vi "InitializeInstrument.vi"(8 "error in (no error)":errorcluster, 11 "reference in":refnum<class "niMmWave_Transceiver.lvclass">) -> (0 "error out":errorcluster, 3 "reference out":refnum<class "niMmWave_Transceiver.lvclass">)   [LabVIEW 2019, in "niMmWave_Transceiver.lvclass"]
doc: "Opens instrument session(s) and performs initial configuration for selected mode.\n\nInputs:\n<b>Initialization source</b> ini file and ini section to be read\n<b>Mode</b> specifies operation mode: BB/IF/RF"
uses:
  niMmWave_Transceiver.lvclass
  C:/Barkhausen mmWave radar/Development/modules/mmw_instrument/src_LabVIEW/Host/SubVIs/mmWave instrument_class/mmWave instrument.lvclass
  Low-level/TypeDefs/Resources.ctl
  <vilib>/userdefined/High Color/nirio_resource_hc.ctl
  mmWave instrument_class/Instrument state.ctl
  Low-level/TypeDefs/Hardware Configuration.ctl
  Low-level/TypeDefs/Direction.ctl
  mmWave HW Control/mmWave HW Control.lvlib
  mmWave instrument_class/mmWave instrument.lvclass
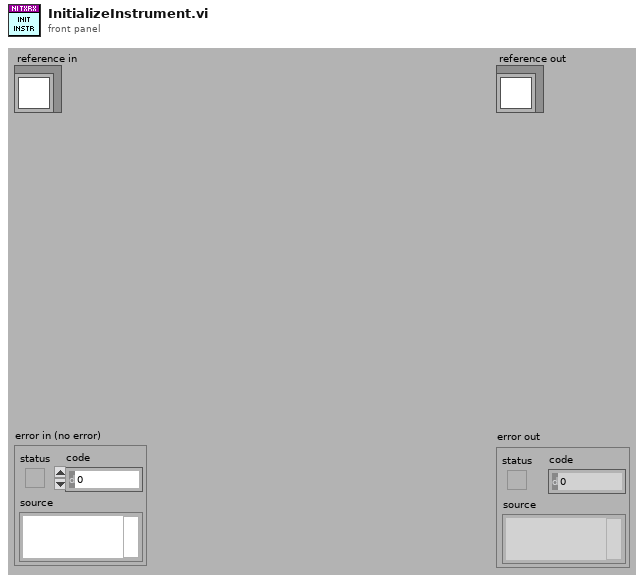
[diagram p1: front panel]
types:
  T1 = typedef "mmWave instrument.lvclass/Instrument state.ctl" = enum16{"Off", "Initialization", "Configuration", "Running", "Calibration"}
  T2 = typedef "Resources.ctl" = cluster{"7902R (Tx)":T3, "3610 (Tx)":refnum<visa-resource-name>, "3620 (IF)":T3, "3630 (RX)":refnum<visa-resource-name>, "7902R (Rx)":T3}
  T3 = typedef "nirio_resource_hc.ctl" = tag
  T4 = typedef "mmWave instrument.lvclass/ObjectAttributesRef.ctl" = refnum<data-value>
  T5 = typedef "niMmWave_Transceiver.lvclass/ObjectAttributesRef.ctl" = refnum<data-value>
  T6 = typedef "niMmWave_Transceiver.lvclass/ObjectAttributes.ctl" = cluster{"session":T7[], "HW.RX resources":T21, "RF config":T22, "RX trigger options":T23, "TX trigger options":T23, "RX samples":i32, "Downloaded Bursts":map{string, T26}, "TX Fs":dbl, "RX Fs":dbl, "burst sequence":string[]}
  T7 = typedef "Session.ctl" = cluster{"3620 session":refnum<queue>, "tx baseband session":T8, "rx baseband session":T16, "tx gain (dB)":dbl, "rx gain (dB)":dbl, "hardware configuration":T17, "gain ranging":T19[], "pxi trigger bus information":T20}
  T8 = typedef "Tx Baseband Session.ctl" = cluster{"3610 session":T9, "7902 reference":T15}
  T9 = typedef "ni3610_and_ni3630_Driver_Lib.lvlib/Main Settings.ctl" = cluster{"VISA resource name":refnum<visa-resource-name>, "Address Space":T10, "window_offset":u32, "register_addresses":T11, "required_MM_fpga_version":cluster{"signature":u32, "hardware":u32, "current revision":u32, "oldest revision":u32}, "CPLD Oldest Compat Version ":cluster{"hardware":u32, "CPLD firmware":u32}, "MM_FPGA_image_location":string, "is_init":bool, "card_type":T12, "DacLmkConfigFileName":string, "AdcLmkConfigFileName":string, "AdcConfigFileName":string, "DacConfigFileName_RevA":string, "DacConfigFileName_RevB":string, "Mulde hardware revision":u8, "bypass DAC PLL\n":bool, "IQ Card Revision":T13, "board capability":T14}
  T10 = typedef "VISA Register Access Address Space.ctl" = u16
  T11 = typedef "ni3610_and_ni3630_Driver_Lib.lvlib/Register Adresses.ctl" = cluster{"MM based Registers":cluster{"Revision":u32, "OldestCompatRev":u32, "signature":u32, "scratch":u32, "LedControl":u32, "BoardHwRev":u32, "BoardControl":u32, "ThermalStatus":u32, "BasebandStatus":u32, "BasebandControl":u32, "BasebandAuxSetup":u32, "BasebandAuxStatus":u32, "LmkSyncOutSetup":u32, " AdcSyncOutSetup":u32, " InjSyncOutSetup":u32, " PxiTrig0OutSetup":u32, " PxiTrig1OutSetup":u32, " PxiTrig2OutSetup":u32, " PxiTrig3OutSetup":u32, " PxiTrig4OutSetup":u32, " PxiTrig5OutSetup":u32, " PxiTrig6OutSetup":u32, " PxiTrig7OutSetup":u32}, "CPLD based Registers":cluster{"SlaveSignature":u32, "SlaveRevision":u32, "SlaveOldestCompatRev":u32, "SlaveScratch":u32, "SlaveSetup":u32, "SlaveStatus":u32, "IDacReg_offset":u32, "LMKRegGrp0_offset":u32, "QDacReg_offset":u32, "BrdTempSensorVal":u32, "TempSensorPowerDown":u32, "GPIOReg_offset":u32, "IAdcReg_offset":u32, "QAdcReg_offset":u32, "LMKRegGrp1_offset":u32, "QadcTempSensorVal":u32, "IadcTempSensorVal":u32, "RevisionReg":u32, "VcxoReg":u32, "CpldStatusReg":u32, "PowerReg":u32, "VBiasEnReg":u32, "ExtRefOeReg":u32, "QdacCtrlReg":u32, "QdacStatusReg":u32, "IdacCtrlReg":u32, "IdacStatusReg":u32, "QdacJtagIn":u32, "QdacJtagOut":u32, "IdacJtagIn":u32, "IdacJtagOut":u32, "IqDcSetupReg":u32, "QadcStatusReg":u32, "IadcStatusReg":u32, "BrdSetupReg":u32, "IqDcRevisionReg":u32, "PllStatusReg":u32, "EndpointScratchReg":u32, "AdcSyncCfgReg":u32, "IqCardOpampReg":u32}, "CPLD Register Offset":u32, "MM  Register Offset":u32, " PxiTrig0OutSetup":u32}
  T12 = typedef "ni3610_and_ni3630_Driver_Lib.lvlib/Base Card Type.ctl" = enum16{"unspecified", "ADC", "DAC"}
  T13 = typedef "ni3610_and_ni3630_Driver_Lib.lvlib/IQ Card Revision.ctl" = enum16{"RevA", "RevB", "RevC", "RevD"}
  T14 = typedef "ni3610_and_ni3630_Driver_Lib.lvlib/Board Capability.ctl" = cluster{"baseband sync":enum16{"no baseband sync", "baseband sync"}}
  T15 = typedef "Blank FPGA Reference.ctl" = refnum<k20>
  T16 = typedef "Rx Baseband Session.ctl" = cluster{"3630 session":T9, "7902 reference":T15}
  T17 = typedef "Hardware Configuration.ctl" = cluster{"direction":T18, "baseband only":bool}
  T18 = typedef "Direction.ctl" = enum16{"Transceiver", "Receiver", "Transmitter"}
  T19 = typedef "Gain Ranging.ctl" = cluster{"gain ranging active scope":string, "gain ranging stream session":refnum<k20>}
  T20 = typedef "PXI Trigger Bus Info.ctl" = cluster{"chassis resource name":refnum<visa-resource-name>, "7902R (TX)":i16, "3610 (TX)":i16, "3620 (IF)":i16, "3630 (RX)":i16, "7902R (RX)":i16}
  T21 = typedef "mmWave HW Control.lvlib/HW TXRX resources cluster.ctl" = cluster{"TX_DAC":refnum<visa-resource-name>, "TX_FPGA":tag, "IF":tag, "RX_ADC":refnum<visa-resource-name>, "RX_FPGA":tag}
  T22 = typedef "mmWave HW Control.lvlib/HW TXRX RF config cluster.ctl" = cluster{"TX.Frequency":dbl, "TX.Gain":dbl, "TX.mmWave adapter":string, "RX.Frequency":dbl, "RX.Gain":dbl, "RX.mmWave adapter":string}
  T23 = typedef "TX trigger config.ctl" = cluster{"delay":dbl, "trig source":T24, "PXI src":i32, "export":T25, "PXI dest":i32}
  T24 = typedef "FPGA Utility.lvlib/FPGA driver trigger source.ctl" = enum16{"Use Tclk", "PXI_Trig", "Aurora RX trig"}
  T25 = typedef "FPGA Utility.lvlib/FPGA driver trigger destination.ctl" = enum16{"None", "Source trig", "Synced trig", "Delayed sync"}
  T26 = typedef "niMmWave_Transceiver.lvclass/BurstInfo.ctl" = cluster{"starting addr":u32, "end addr":u32}
  T27 = typedef "mmWave instrument.lvclass/ObjectAttributes.ctl" = cluster{"mode":T28, "instr state":T1, "Max Fs":dbl, "Equalization coeff":cdb[], "LO sync en":bool, "Trig sync en":bool, "LO sources":T29, "LO Export":T30, "Fc.range":cluster{"min":dbl, "max":dbl}, "Sync mode":T31, "equalization en":bool, "sequence":string[]}
  T28 = typedef "mmWave instrument.lvclass/Instrument mode.ctl" = enum16{"RF", "IF", "BB"}
  T29 = typedef "mmWave HW Control.lvlib/LO sources.ctl" = cluster{"RX/LO1 src":string, "TX/LO1 src":string, "LO2 src":string}
  T30 = typedef "mmWave HW Control.lvlib/LO export.ctl" = cluster{"TX LO1 export":bool, "TX LO1 export level":dbl, "RX LO1 export":bool, "RX LO1 export level":dbl, "LO2 export":bool, "LO2 export level":dbl}
  T31 = typedef "mmWave instrument.lvclass/Sync mode.ctl" = enum16{"Slave", "Master"}
  T32 = typedef "Detected mmWave Adapters.ctl" = cluster{"3620 resource name":T3, "detected mmWave adapters":T33[]}
  T33 = typedef "mmWave Adapter Information.ctl" = cluster{"scope":string, "mmWave adapter type":string, "serial number":u64}
  T34 = typedef "Constants.ctl" = cluster{"data clock rate (Hz)":dbl, "sample rate (Hz)":dbl, "sample rate selector string":string, "default tx bitfile path":path, "default rx bitfile path":path, "default proc bitfile path":path}
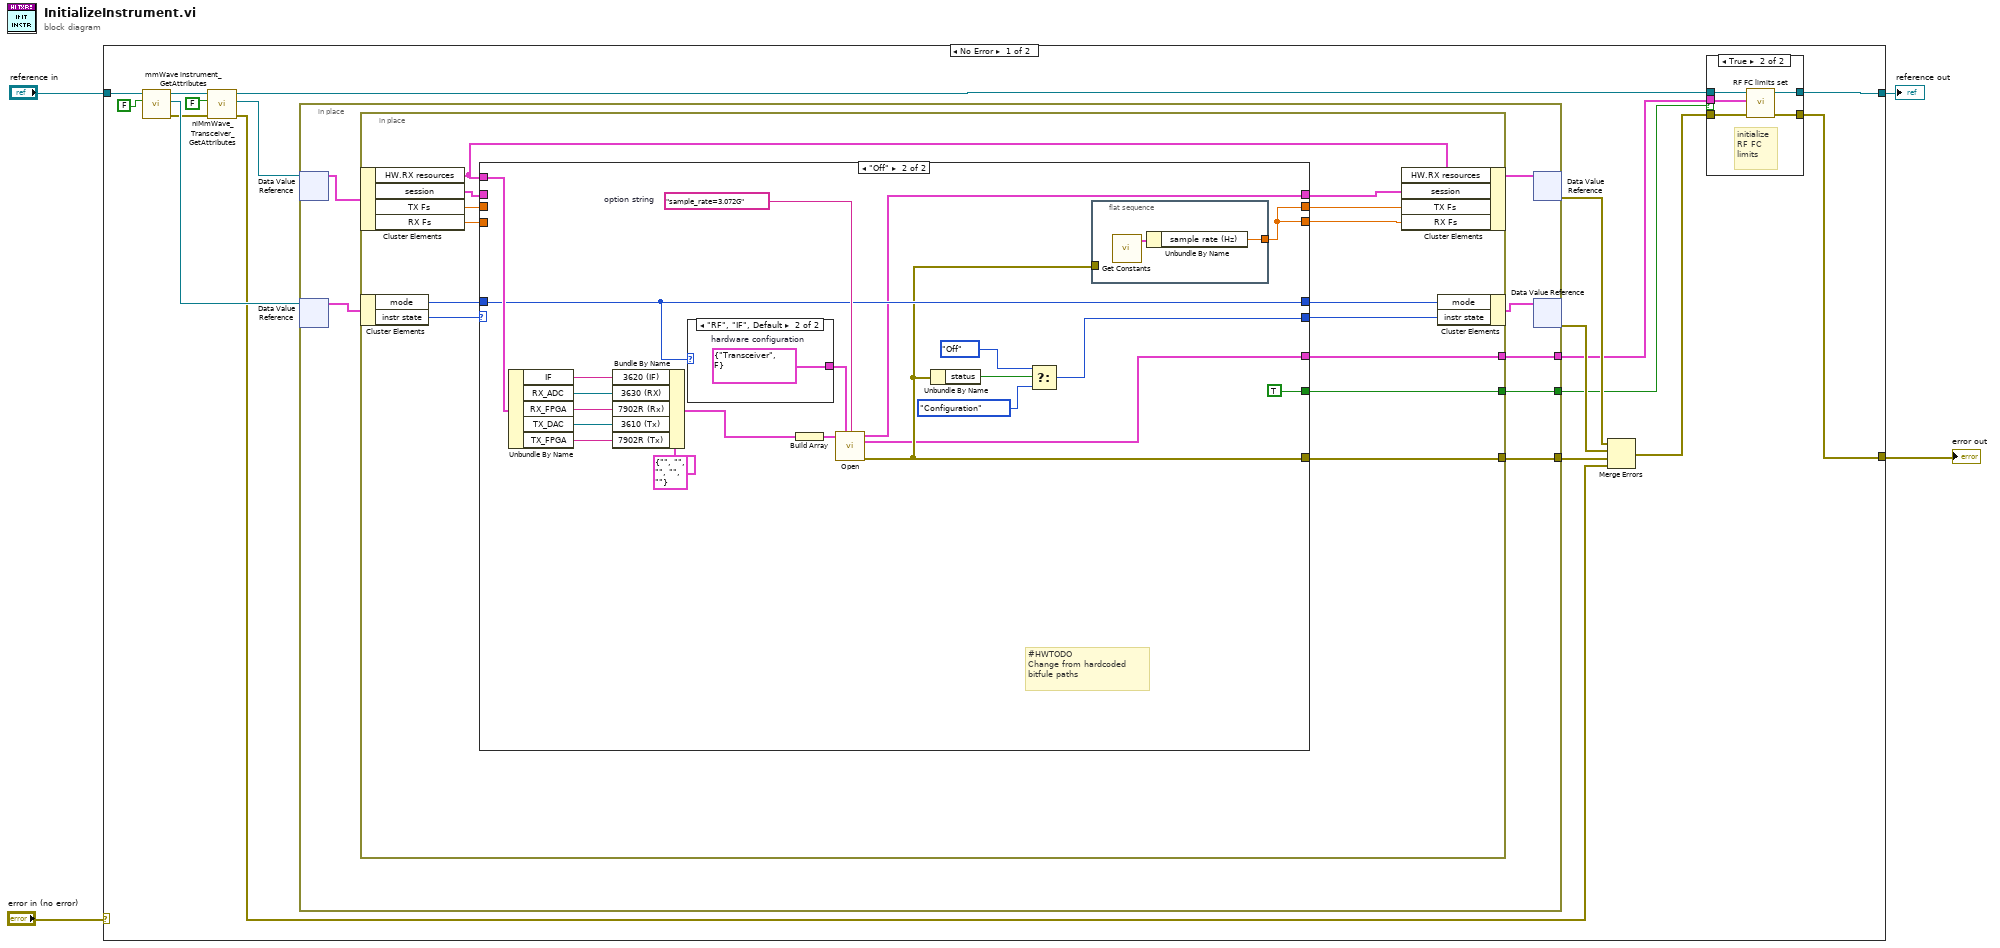
[diagram p0: block diagram]
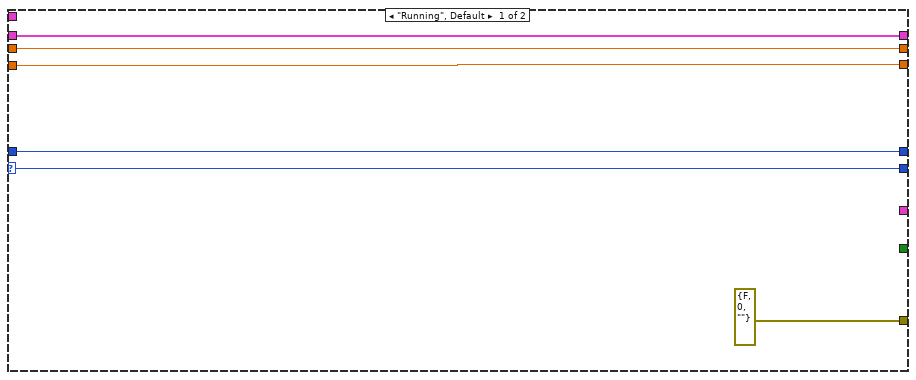
[diagram p3: hidden frame]
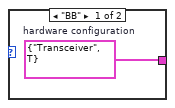
[diagram p4: hidden frame]
diagram:
  n1 = case shown="No Error" "error in (no error)" {
    selector: "error in (no error)" -> [_ w82]
    tunnel: [w6 w82] -> w3
    tunnel: [w9 w81] -> w1
    tunnel: "reference in" -> [w20 w81]
    frame No Error {
      n2 = call "mmWave instrument_GetAttributes.vi"("return data? (T)"=FALSE, "reference in"=w20) -> ("error out"=w13:errorcluster, "attributes ref"=w15:T4, "reference out"=w19:refnum<class "niMmWave_Transceiver.lvclass">)  [unwired: 6 in, 1 out]
      n3 = call "niMmWave_Transceiver_GetAttributes.vi"("error in (no error)"=w13, "return data? (T)"=FALSE, "reference in"=w19) -> ("error out"=w10:errorcluster, "attributes ref"=w16:T5, "reference out"=w21:refnum<class "niMmWave_Transceiver.lvclass">)  [unwired: 5 in, 1 out]
      n4 = in-place {
        in-place-border: [w31] -> w14
        in-place-border: [w30] -> w8
        in-place-border: [w29] -> w5
        n5 = in-place-dvr #1(w16) -> (w35:T6)  [unwired: 1 out]
        n6 = in-place-dvr #2(w15) -> (w33:T27)  [unwired: 1 out]
        n7 = in-place {
          in-place-border: [w46] -> w31
          in-place-border: [w38] -> w30
          in-place-border: [w37] -> w29
          n8 = in-place-cluster #3(w35) -> ("HW.RX resources"=w49:T21, "session"=w36:T7[], "TX Fs"=w40:dbl, "RX Fs"=w39:dbl)
          n9 = in-place-cluster #4(w33) -> ("mode"=w47:T28, "instr state"=w44:T1)
          n10 = case shown="\"Off\"" w44 {
            selector: w44 -> [w50 _]
            tunnel: w49 -> [_ w67]
            tunnel: [w51 w58] -> w48
            tunnel: w47 -> [w55 w61]
            tunnel: [errorcluster {"status"=FALSE, "code"=0, "source"=""} ("error out") w60] -> w46
            tunnel: [w50 w62] -> w45
            tunnel: [w55 w61] -> w43
            tunnel: [w53 w59] -> w42
            tunnel: [w52 w59] -> w41
            tunnel: w40 -> [w53 _]
            tunnel: w39 -> [w52 _]
            tunnel: [_ w57] -> w38
            tunnel: [_ TRUE] -> w37
            tunnel: w36 -> [w51 _]
            frame "Running", Default {
            }
            frame "Off" {
              w70 = "sample_rate=3.072G"  # option string
              # "#HWTODO\nChange from hardcoded\nbitfule paths"
              n11 = Unbundle By Name(w67) -> ("IF"=w74:tag, "RX_ADC"=w73:refnum<visa-resource-name>, "RX_FPGA"=w72:tag, "TX_DAC"=w69:refnum<visa-resource-name>, "TX_FPGA"=w68:tag)
              n12 = Bundle By Name(cluster=T2 {"7902R (Tx)"="", "3610 (Tx)"="", "3620 (IF)"="", "3630 (RX)"="", "7902R (Rx)"=""} ("resources"), "3620 (IF)"=w74, "3630 (RX)"=w73, "7902R (Rx)"=w72, "3610 (Tx)"=w69, "7902R (Tx)"=w68) -> (w76:T2)
              n13 = case shown="\"RF\", \"IF\", Default" w61 {
                tunnel: [w79 w80] -> w66
                frame "BB" {
                  w79 = T17 {"direction"=enum."Transceiver", "baseband only"=TRUE}  # hardware configuration
                }
                frame "RF", "IF", Default {
                  w80 = T17 {"direction"=enum."Transceiver", "baseband only"=FALSE}  # hardware configuration
                }
              }
              n14 = Build Array(w76) -> (w75:T2[])
              n15 = call "Open.vi"("resources"=w75, "hardware configuration"=w66, "option string"=w70) -> ("session out"=w58:T7[], "detected mmWave adapters"=w57:T32[], "error out"=w60:errorcluster)  [unwired: 10 in]
              n16 = Unbundle By Name(w60) -> ("status"=w65:bool)
              n17 = Select(t=Instrument_state."Off" ("instr state"), s=w65, f=Instrument_state."Configuration" ("instr state")) -> (s? t:f=w62:T1)
              n18 = flat-sequence {
                tunnel: w60 -> [_]
                tunnel: [w78] -> w59
                frame #0 {
                  n19 = call "Get Constants.vi"() -> ("constants"=w77:T34)  [unwired: 15 in]
                  n20 = Unbundle By Name(w77) -> ("sample rate (Hz)"=w78:dbl)
                }
              }
            }
          }
          n21 = in-place-cluster #3("HW.RX resources"=w49, "session"=w48, "TX Fs"=w42, "RX Fs"=w41) -> (w34:T6)
          n22 = in-place-cluster #4("mode"=w43, "instr state"=w45) -> (w32:T27)
        }
        n23 = in-place-dvr #1(w34) -> (w12:errorcluster)  [unwired: 1 out]
        n24 = in-place-dvr #2(w32) -> (w11:errorcluster)  [unwired: 1 out]
      }
      n25 = Merge Errors(w12, w11, w14, w10) -> (w7:errorcluster)
      n26 = case shown="True" w5 {
        tunnel: w21 -> [w23 w28]
        tunnel: [w23 w27] -> w9
        tunnel: w8 -> [_ w26]
        tunnel: w7 -> [w22 w25]
        tunnel: [w22 w24] -> w6
        frame False {
        }
        frame True {
          # "initialize\nRF FC \nlimits"
          n27 = call-dynamic "RF FC limits set.vi"("error in (no error)"=w25, "detected mmWave adapters"=w26, "reference in"=w28) -> ("error out"=w24:errorcluster, "reference out"=w27:refnum<class "niMmWave_Transceiver.lvclass">)  [unwired: 7 in]
        }
      }
    }
    frame Error {
    }
  }
  "error out" <- w3
  "reference out" <- w1
